vi "Multiple Random Numbers.vi"(11 "No. of rands":i32=2) -> (3 "Random numbers":dbl[](array[numeric]))   [LabVIEW 2014, in "HMM.lvlib"]
doc: "Generates multiple random numbers, the sum of which is equal to 1."
uses:
  HMM.lvlib
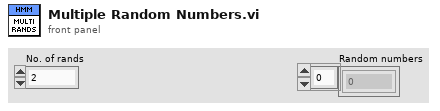
[diagram p1: front panel]
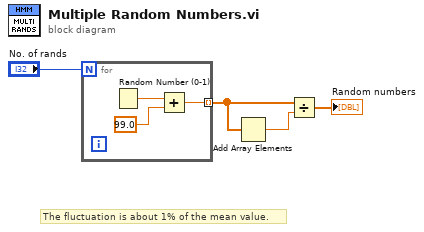
[diagram p0: block diagram]
diagram:
  # "The fluctuation is about 1% of the mean value."
  n1 = for {
    N: "No. of rands" -> [_]
    tunnel: [w6] -> w3 mode=indexing
    n2 = Random Number (0-1)() -> (number: 0 to 1=w7:dbl)
    n3 = Add(x=w7, y=99.0) -> (x+y=w6:dbl)
  }
  n4 = Add Array Elements(numeric array=w3) -> (sum=w2:dbl)
  n5 = Divide(x=w3, y=w2) -> (x/y=→"Random numbers":dbl[])
